vi "pressure max.vi"(0 "unsigned byte array":u8[](array[numeric])) -> (10 "x-y 9":dbl, 11 "x-y 10":dbl, 12 "x-y 7":dbl, 13 "x-y 8":dbl, 14 "x-y 1":dbl, 15 "x-y 2":dbl, 16 "x-y 3":dbl, 17 "x-y 4":dbl, 18 "x-y 5":dbl, 19 "x-y 6":dbl)   [LabVIEW 2016]
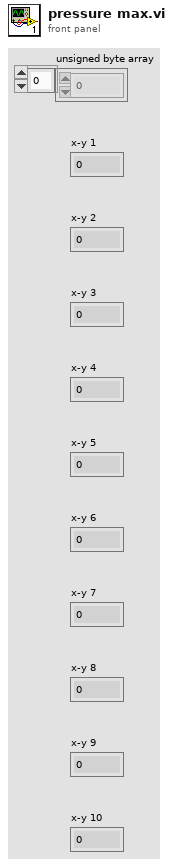
[diagram p1: front panel]
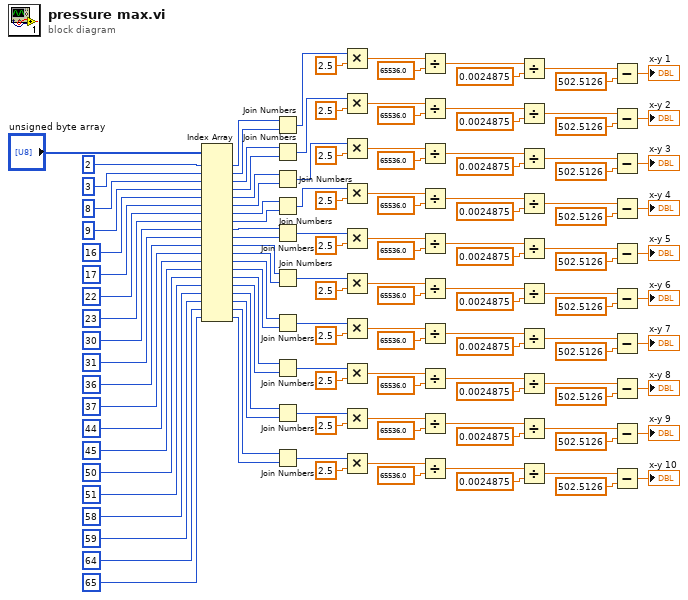
[diagram p0: block diagram]
diagram:
  n1 = Index Array(array="unsigned byte array", index #1=2 ("index"), index #2=3 ("index"), index #3=8 ("index"), index #4=9 ("index"), index #5=16 ("index"), index #6=17 ("index"), index #7=22 ("index"), index #8=23 ("index"), index #9=30 ("index"), index #10=31 ("index"), index #11=36 ("index"), index #12=37 ("index"), index #13=44 ("index"), index #14=45 ("index"), index #15=50 ("index"), index #16=51 ("index"), index #17=58 ("index"), index #18=59 ("index"), index #19=64 ("index"), index #20=65 ("index")) -> (element #1=w112:u8, element #2=w113:u8, element #3=w114:u8, element #4=w115:u8, element #5=w116:u8, element #6=w117:u8, element #7=w118:u8, element #8=w119:u8, element #9=w120:u8, element #10=w121:u8, element #11=w122:u8, element #12=w123:u8, element #13=w124:u8, element #14=w125:u8, element #15=w126:u8, element #16=w127:u8, element #17=w128:u8, element #18=w129:u8, element #19=w130:u8, element #20=w131:u8)
  n2 = Join Numbers(hi=w112, lo=w113) -> ((hi.lo)=w9:u16)
  n3 = Join Numbers(hi=w114, lo=w115) -> ((hi.lo)=w8:u16)
  n4 = Join Numbers(hi=w116, lo=w117) -> ((hi.lo)=w7:u16)
  n5 = Join Numbers(hi=w118, lo=w119) -> ((hi.lo)=w6:u16)
  n6 = Join Numbers(hi=w120, lo=w121) -> ((hi.lo)=w5:u16)
  n7 = Join Numbers(hi=w122, lo=w123) -> ((hi.lo)=w4:u16)
  n8 = Join Numbers(hi=w124, lo=w125) -> ((hi.lo)=w3:u16)
  n9 = Join Numbers(hi=w126, lo=w127) -> ((hi.lo)=w2:u16)
  n10 = Join Numbers(hi=w128, lo=w129) -> ((hi.lo)=w1:u16)
  n11 = Join Numbers(hi=w130, lo=w131) -> ((hi.lo)=w83:u16)
  n12 = Multiply(x=w9, y=2.5) -> (x*y=w80:dbl)
  n13 = Multiply(x=w8, y=2.5) -> (x*y=w72:dbl)
  n14 = Multiply(x=w7, y=2.5) -> (x*y=w64:dbl)
  n15 = Multiply(x=w6, y=2.5) -> (x*y=w56:dbl)
  n16 = Multiply(x=w5, y=2.5) -> (x*y=w48:dbl)
  n17 = Multiply(x=w4, y=2.5) -> (x*y=w40:dbl)
  n18 = Multiply(x=w3, y=2.5) -> (x*y=w32:dbl)
  n19 = Multiply(x=w2, y=2.5) -> (x*y=w24:dbl)
  n20 = Multiply(x=w1, y=2.5) -> (x*y=w16:dbl)
  n21 = Multiply(x=w83, y=2.5) -> (x*y=w89:dbl)
  n22 = Divide(x=w80, y=65536.0) -> (x/y=w78:dbl)
  n23 = Divide(x=w72, y=65536.0) -> (x/y=w70:dbl)
  n24 = Divide(x=w64, y=65536.0) -> (x/y=w62:dbl)
  n25 = Divide(x=w56, y=65536.0) -> (x/y=w54:dbl)
  n26 = Divide(x=w48, y=65536.0) -> (x/y=w46:dbl)
  n27 = Divide(x=w40, y=65536.0) -> (x/y=w38:dbl)
  n28 = Divide(x=w32, y=65536.0) -> (x/y=w30:dbl)
  n29 = Divide(x=w24, y=65536.0) -> (x/y=w22:dbl)
  n30 = Divide(x=w16, y=65536.0) -> (x/y=w14:dbl)
  n31 = Divide(x=w89, y=65536.0) -> (x/y=w87:dbl)
  n32 = Divide(x=w78, y=0.0024875) -> (x/y=w81:dbl)
  n33 = Divide(x=w70, y=0.0024875) -> (x/y=w73:dbl)
  n34 = Divide(x=w62, y=0.0024875) -> (x/y=w65:dbl)
  n35 = Divide(x=w54, y=0.0024875) -> (x/y=w57:dbl)
  n36 = Divide(x=w46, y=0.0024875) -> (x/y=w49:dbl)
  n37 = Divide(x=w38, y=0.0024875) -> (x/y=w41:dbl)
  n38 = Divide(x=w30, y=0.0024875) -> (x/y=w33:dbl)
  n39 = Divide(x=w22, y=0.0024875) -> (x/y=w25:dbl)
  n40 = Divide(x=w14, y=0.0024875) -> (x/y=w17:dbl)
  n41 = Divide(x=w87, y=0.0024875) -> (x/y=w90:dbl)
  n42 = Subtract(x=w81, y=502.5126) -> (x-y=→"x-y 1":dbl)
  n43 = Subtract(x=w73, y=502.5126) -> (x-y=→"x-y 2":dbl)
  n44 = Subtract(x=w65, y=502.5126) -> (x-y=→"x-y 3":dbl)
  n45 = Subtract(x=w57, y=502.5126) -> (x-y=→"x-y 4":dbl)
  n46 = Subtract(x=w49, y=502.5126) -> (x-y=→"x-y 5":dbl)
  n47 = Subtract(x=w41, y=502.5126) -> (x-y=→"x-y 6":dbl)
  n48 = Subtract(x=w33, y=502.5126) -> (x-y=→"x-y 7":dbl)
  n49 = Subtract(x=w25, y=502.5126) -> (x-y=→"x-y 8":dbl)
  n50 = Subtract(x=w17, y=502.5126) -> (x-y=→"x-y 9":dbl)
  n51 = Subtract(x=w90, y=502.5126) -> (x-y=→"x-y 10":dbl)
